vi "reverseDrive.vi"(9 "Throttle Input":dbl, 10 "Toggle Input":dbl) -> (2 "Final Throttle Value":dbl, 6 "reverseDrive?":bool)   [LabVIEW 2017]
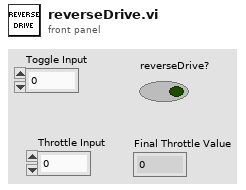
[diagram p1: front panel]
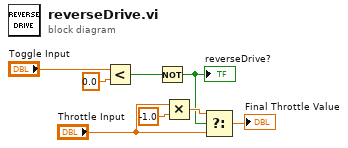
[diagram p0: block diagram]
diagram:
  n1 = Less?(x="Toggle Input", y=0.0) -> (x < y?=w2:bool)
  n2 = Not(x=w2) -> (.not. x?=w1:bool)
  "reverseDrive?" <- w1
  n3 = Multiply(x="Throttle Input", y=-1.0) -> (x*y=w4:dbl)
  n4 = Select(t=w4, s=w1, f="Throttle Input") -> (s? t:f=→"Final Throttle Value":dbl)
